vi "Prod-Cons-UI.vi"() -> ()   [LabVIEW 2024]
uses:
  TypeDefs/Messages.ctl
panel:
  out "Komunikaty":string
  out "HistoryGraph":cluster{"X":dbl, "Y":dbl}[](graph)
  out "unit":string
  out "timestamp":u64
  out "value":dbl
  out "sensor":string
  out "device_id":string
  in  "History":bool
  in  "Latest":bool
  in  "Limit":i32
  in  "Sensors":u16(ring) items=["temp", "hum", "pressure"]
  in  "Device":u16(ring) items=["esp32-abcd01", "esp32-abcd03", "esp32-abcd02"]
  in  "Refresh Interval":i32
  in  "Auto Refresh":bool
  in  "Refresh":bool
  in  "Test API":bool
  out "StatusAPI":string
  in  "API-URL":string
  in  "stop":bool
  # "Rozproszone Systemy Pomiarowe - Dasboard LabVIEW"
  # "REST API URL:"
  # "Status API:"
  # "Konfiguracja i filtry"
  # "Device"
  # "Sensor"
  # "Limit"
  # "Latest measurement"
  # "Device ID"
  # "Sensor"
  # "Value"
  # "Unit"
  # "TimeStamp"
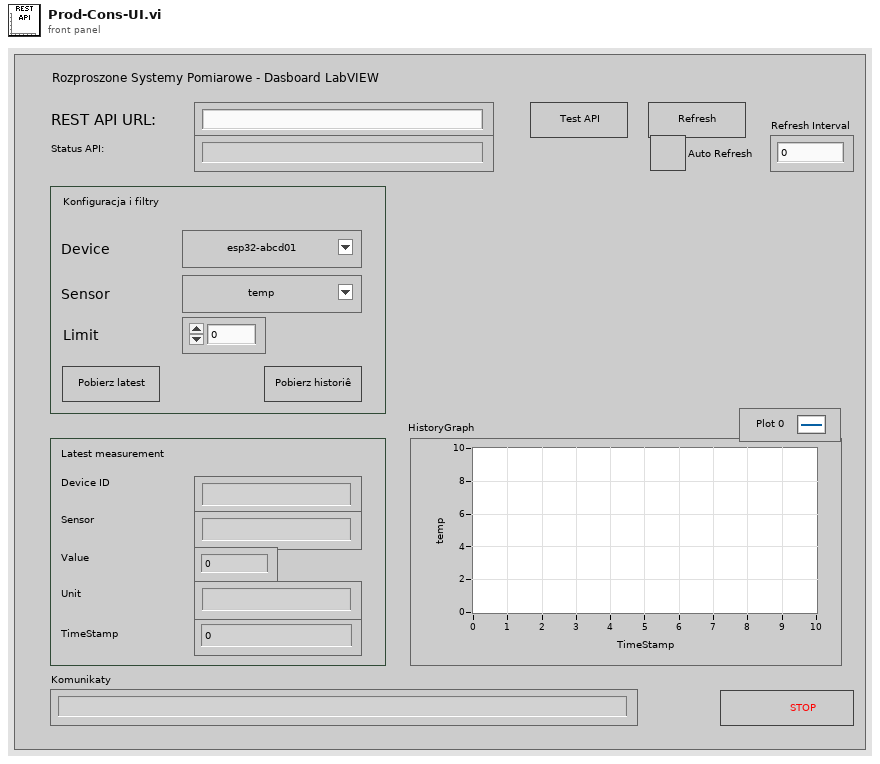
[diagram p1: front panel]
types:
  T1 = typedef "Messages.ctl" = cluster{"CMD":enum16{"Init", "Stop", "TestAPI", "Refresh", "Latest", "History", "LoadDevices"}, "Parameter":variant}
  T2 = enum16{"Init", "Stop", "TestAPI", "Refresh", "Latest", "History", "LoadDevices"}
  T3 = typedef "MeasurementData.ctl" = cluster{"device_id":string, "sensor":string, "value":dbl, "unit":string, "group_id":string}
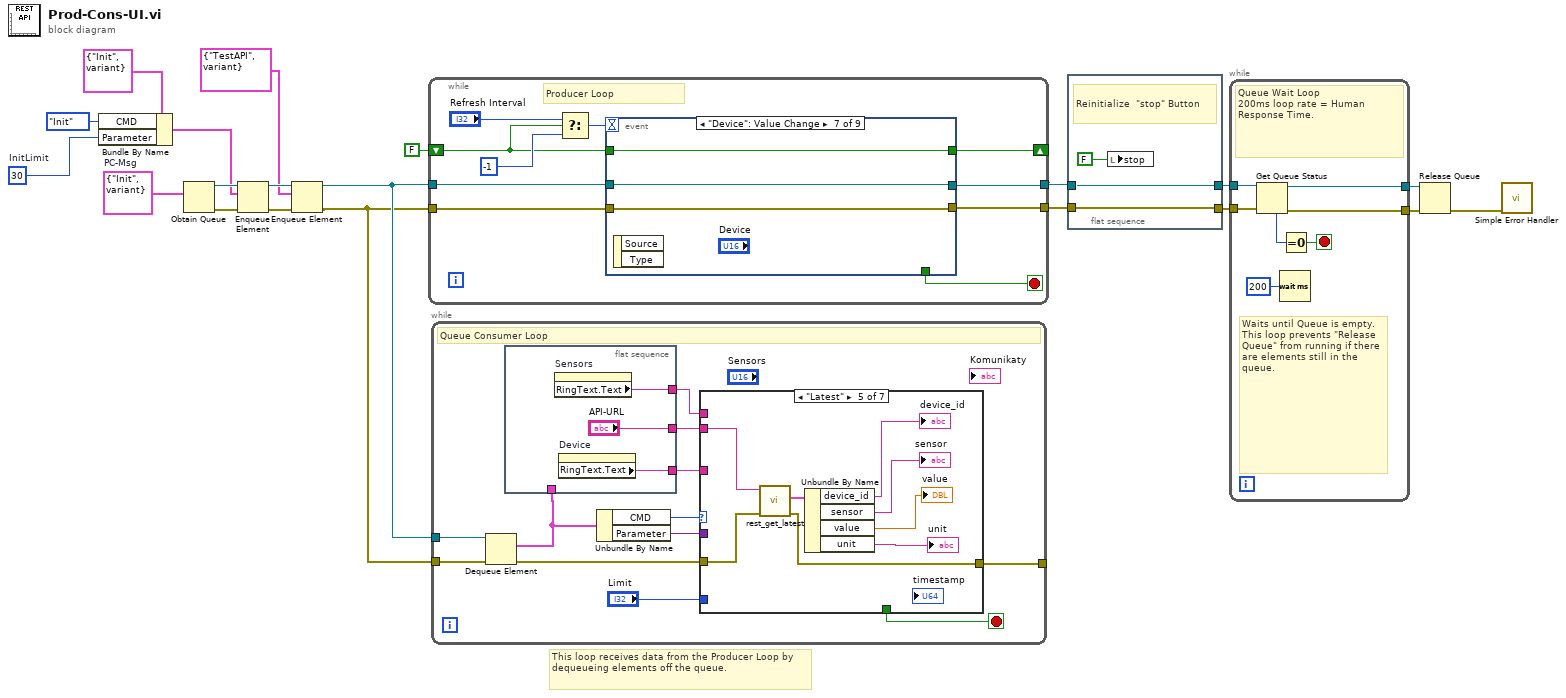
[diagram p0: block diagram]
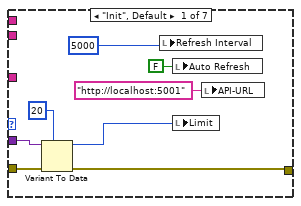
[diagram p2: hidden frame]
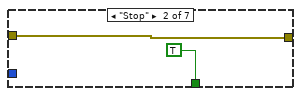
[diagram p3: hidden frame]
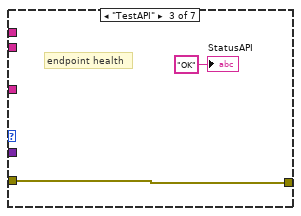
[diagram p4: hidden frame]
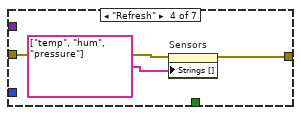
[diagram p5: hidden frame]
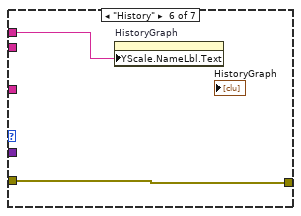
[diagram p6: hidden frame]
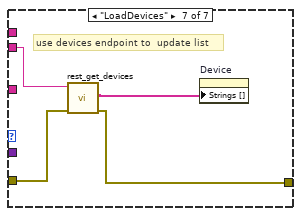
[diagram p7: hidden frame]
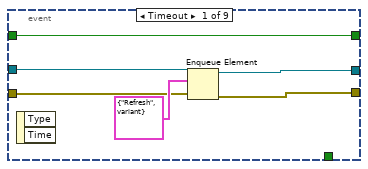
[diagram p8: hidden frame]
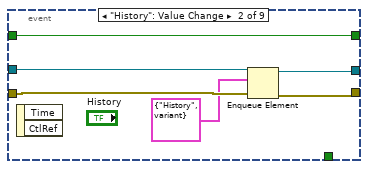
[diagram p9: hidden frame]
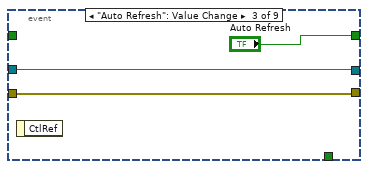
[diagram p10: hidden frame]
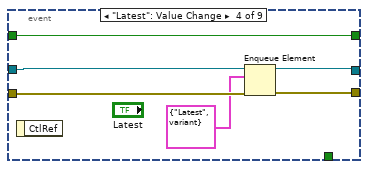
[diagram p11: hidden frame]
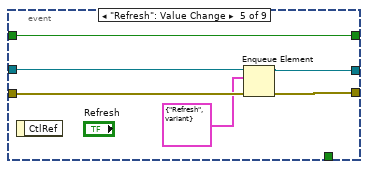
[diagram p12: hidden frame]
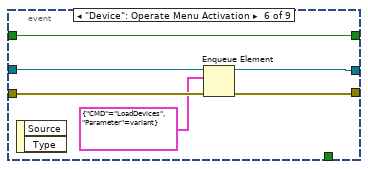
[diagram p13: hidden frame]
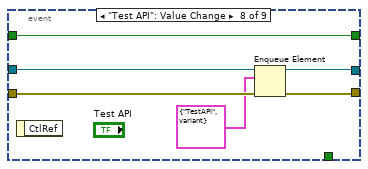
[diagram p14: hidden frame]
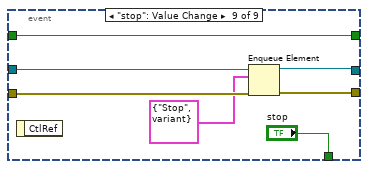
[diagram p15: hidden frame]
diagram:
  w9 = 30  # InitLimit
  w15 = T1 {"CMD"=enum."Init", "Parameter"=variant}  # PC-Msg
  # "This loop receives data from the Producer Loop by dequeueing elements off the queue."
  n1 = Bundle By Name(cluster=T1 {"CMD"=enum."Init", "Parameter"=variant} ("element"), "CMD"=enum16{"Init", "Stop", "TestAPI"}."Init", "Parameter"=w9) -> (w8:T1)
  n2 = Obtain Queue(element data type=w15) -> (queue out=w14:refnum<queue>, error out=w12:errorcluster)  [unwired: 4 in, 1 out]
  n3 = Enqueue Element(queue=w14, element=w8, error in (no error)=w12) -> (queue out=w13:refnum<queue>, error out=w3:errorcluster)  [unwired: 2 out]
  n4 = Enqueue Element(queue=w13, element=T1 {"CMD"=enum."TestAPI", "Parameter"=variant}, error in (no error)=w3) -> (queue out=w4:refnum<queue>, error out=w2:errorcluster)  [unwired: 1 in, 1 out]
  n5 = while {
    tunnel: w4 -> [w27]
    tunnel: w2 -> [w24]
    tunnel: [w22] -> w17
    shift-right: [w26] -> _
    shift-left: FALSE ("Auto Refresh") -> [w21]
    tunnel: [w23] -> w6
    stop <- w30 stop-if-true
    # "Producer Loop"
    n6 = Select(t="Refresh Interval", s=w21, f=-1) -> (s? t:f=w25:i32)
    n7 = event shown="[6] \"Device\": Value Change" {
      selector: _ -> [_ _ _ _ _ _ _ _ _]
      dyn-events: _ -> [_ _ _ _ _ _ _ _ _]
      timeout: w25 -> [_ _ _ _ _ _ _ _ _]
      tunnel: [_ _ _ _ _ _ _ _ "stop"] -> w30
      tunnel: w27 -> [w36 w42 w45 w51 w56 w62 w66 w72 w78]
      tunnel: [w33 w39 w45 w50 w55 w61 w66 w71 w75] -> w22
      tunnel: [w31 w37 "Auto Refresh" w46 w52 w63 w65 w67 w73] -> w26
      tunnel: w24 -> [w34 w41 w43 w49 w57 w60 w64 w70 w77]
      tunnel: [w32 w40 w43 w48 w54 w59 w64 w69 w76] -> w23
      tunnel: w21 -> [w31 w37 _ w46 w52 w63 w65 w67 w73]
      event Timeout {
        n8 = event-data() -> ()  [unwired: 1 in, 2 out]
        n9 = Enqueue Element(queue=w36, element=T1 {"CMD"=enum."Refresh", "Parameter"=variant}, error in (no error)=w34) -> (queue out=w33:refnum<queue>, error out=w32:errorcluster)  [unwired: 2 out]
      }
      event "History": Value Change {
        n10 = event-data() -> ()  [unwired: 1 in, 2 out]
        n11 = Enqueue Element(queue=w42, element=T1 {"CMD"=enum."History", "Parameter"=variant}, error in (no error)=w41) -> (queue out=w39:refnum<queue>, error out=w40:errorcluster)  [unwired: 2 out]
      }
      event "Auto Refresh": Value Change {
        n12 = event-data() -> ()  [unwired: 1 in, 1 out]
      }
      event "Latest": Value Change {
        n13 = event-data() -> ()  [unwired: 1 in, 1 out]
        n14 = Enqueue Element(queue=w51, element=T1 {"CMD"=enum."Latest", "Parameter"=variant}, error in (no error)=w49) -> (queue out=w50:refnum<queue>, error out=w48:errorcluster)  [unwired: 2 out]
      }
      event "Refresh": Value Change {
        n15 = event-data() -> ()  [unwired: 1 in, 1 out]
        n16 = Enqueue Element(queue=w56, element=T1 {"CMD"=enum."Refresh", "Parameter"=variant}, error in (no error)=w57) -> (queue out=w55:refnum<queue>, error out=w54:errorcluster)  [unwired: 2 out]
      }
      event "Device": Operate Menu Activation {
        n17 = event-data() -> ()  [unwired: 1 in, 2 out]
        n18 = Enqueue Element(queue=w62, element=T1 {"CMD"=enum."LoadDevices", "Parameter"=variant}, error in (no error)=w60) -> (queue out=w61:refnum<queue>, error out=w59:errorcluster)  [unwired: 2 out]
      }
      event "Device": Value Change {
        n19 = event-data() -> ()  [unwired: 1 in, 2 out]
      }
      event "Test API": Value Change {
        n20 = event-data() -> ()  [unwired: 1 in, 1 out]
        n21 = Enqueue Element(queue=w72, element=T1 {"CMD"=enum."TestAPI", "Parameter"=variant}, error in (no error)=w70) -> (queue out=w71:refnum<queue>, error out=w69:errorcluster)  [unwired: 2 out]
      }
      event "stop": Value Change {
        n22 = event-data() -> ()  [unwired: 1 in, 1 out]
        n23 = Enqueue Element(queue=w78, element=T1 {"CMD"=enum."Stop", "Parameter"=variant}, error in (no error)=w77) -> (queue out=w75:refnum<queue>, error out=w76:errorcluster)  [unwired: 2 out]
      }
    }
  }
  n24 = while {
    tunnel: w4 -> [w91]
    tunnel: w2 -> [w90]
    tunnel: [w86] -> _
    stop <- w87 stop-if-true
    # "Queue Consumer Loop"
    n25 = Dequeue Element(queue=w91, error in (no error)=w90) -> (element=w81:T1, error out=w88:errorcluster)  [unwired: 3 out]
    n26 = flat-sequence {
      tunnel: [w94] -> w85
      tunnel: ["API-URL"] -> w84
      tunnel: [w92] -> w83
      tunnel: w81 -> [_]
      frame #0 {
        n27 = property on="Sensors" class="Ring (strict)"() -> ("RingText.Text"=w94:string)  [unwired: 2 in, 2 out]
        n28 = property on="Device" class="Ring (strict)"() -> ("RingText.Text"=w92:string)  [unwired: 2 in, 2 out]
      }
    }
    n29 = Unbundle By Name(w81) -> ("CMD"=w89:T2, "Parameter"=w80:variant)
    n30 = case shown="\"Latest\"" w89 {
      tunnel: w88 -> [w98 w103 w106 w108 w116 w118 w121]
      tunnel: [_ TRUE _ _ _ _ _] -> w87
      tunnel: [w96 w103 w106 w108 w115 w118 w120] -> w86
      tunnel: w85 -> [_ _ _ _ _ w117 _]
      tunnel: w84 -> [_ _ _ _ w114 _ w122]
      tunnel: w83 -> [_ _ _ _ _ _ _]
      tunnel: "Limit" -> [_ _ _ _ _ _ _]
      tunnel: w80 -> [w99 _ _ _ _ _ _]
      frame "Init", Default {
        n31 = Variant To Data(error in=w98, type=20 ("Limit"), Variant=w99) -> (data=w95:i32, error out=w96:errorcluster)
        n32 = local write "Refresh Interval"(5000 ("Refresh Interval")) -> ()
        n33 = local write "Auto Refresh"(FALSE ("Auto Refresh")) -> ()
        n34 = local write "Limit"(w95) -> ()
        n35 = local write "API-URL"("http://localhost:5001" ("API-URL")) -> ()
      }
      frame "Stop" {
      }
      frame "TestAPI" {
        # "endpoint health"
        "StatusAPI" <- "OK" ("StatusAPI")
      }
      frame "Refresh" {
        n36 = property on="Sensors" class="Ring (strict)"("Strings []"=string[] ["temp", "hum", "pressure"]) -> ()  [unwired: 2 in, 2 out]
      }
      frame "Latest" {
        n37 = call "rest_get_latest.vi"("error in (no error)"=w116, "Base URL"=w114) -> ("error out"=w115:errorcluster, "value"=w113:T3)  [unwired: 8 in]
        n38 = Unbundle By Name(w113) -> ("device_id"=→"device_id":string, "sensor"=→"sensor":string, "value"=→"value":dbl, "unit"=→"unit":string)
      }
      frame "History" {
        n39 = property on="HistoryGraph" class="XYGraph (strict)"("YScale.NameLbl.Text"=w117) -> ()  [unwired: 2 in, 2 out]
      }
      frame "LoadDevices" {
        # "use devices endpoint to  update list"
        n40 = call "rest_get_devices.vi"("error in"=w121, "Base URL"=w122) -> ("error out"=w120:errorcluster, "DeviceArray"=w119:string[])  [unwired: 8 in]
        n41 = property on="Device" class="Ring (strict)"("Strings []"=w119) -> ()  [unwired: 2 in, 2 out]
      }
    }
  }
  n42 = flat-sequence {
    tunnel: w17 -> [w125]
    tunnel: [w125] -> w16
    tunnel: w6 -> [w123]
    tunnel: [w123] -> w5
    frame #0 {
      # "Reinitialize  \"stop\" Button"
      n43 = local write "stop"(FALSE ("stop")) -> ()
    }
  }
  n44 = while {
    tunnel: w16 -> [w132]
    tunnel: [w131] -> w20
    tunnel: [w130] -> w19
    tunnel: w5 -> [w126]
    stop <- w128 stop-if-true
    # "Waits until Queue is empty.  This loop prevents \"Release Queue\" from running if there are elements still in the queue."
    # "Queue Wait Loop\n200ms loop rate = Human Response Time."
    n45 = Get Queue Status(queue=w132, error in (no error)=w126) -> (queue out=w130:refnum<queue>, error out=w131:errorcluster, # elements in queue=w129:i32)  [unwired: 6 out]
    n46 = Wait (ms)(milliseconds to wait=u32 200) -> ()  [unwired: 1 out]
    n47 = Equal To 0?(x=w129) -> (x = 0?=w128:bool)
  }
  n48 = Release Queue(queue=w19, error in (no error)=w20) -> (error out=w18:errorcluster)  [unwired: 3 out]
  n49 = call <vilib>:"Simple Error Handler.vi"("error in (no error)"=w18) -> ()  [unwired: 2 in, 7 out]
